vi "GetControlsAndIndicators.vi"(11 "TopLevelDiagram in":refnum<vi>) -> (2 "All Indicators":refnum<vi>[](array[refnum]), 3 "All ControlsTerminals":refnum<vi>[](array[refnum]))   [LabVIEW 2017]
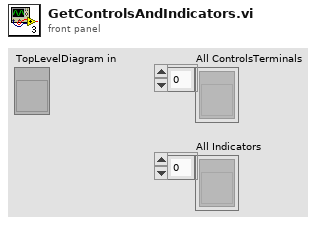
[diagram p1: front panel]
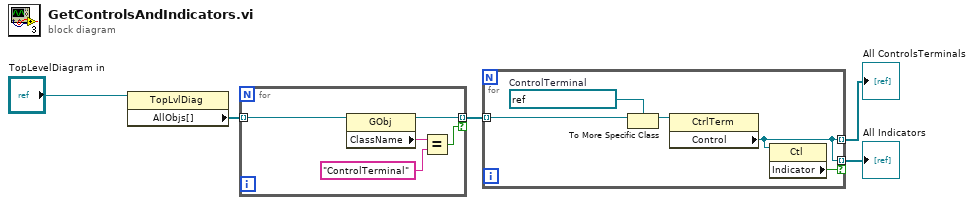
[diagram p0: block diagram]
diagram:
  n1 = property class="TopLvlDiag"(reference="TopLevelDiagram in") -> ("AllObjs[]"=w2:refnum<vi>[])  [unwired: 1 in, 2 out]
  n2 = for {
    tunnel: w2 -> [w10] mode=indexing
    tunnel: [w9] -> w3 mode=indexing if=w6
    n3 = property class="GObj"(reference=w10) -> (reference out=w9:refnum<vi>, "ClassName"=w8:string)  [unwired: 1 in, 1 out]
    n4 = Equal?(x=w8, y="ControlTerminal") -> (x = y?=w6:bool)
  }
  n5 = for {
    tunnel: w3 -> [w15] mode=indexing
    tunnel: [w12] -> w4 mode=indexing
    tunnel: [w12] -> w5 mode=indexing if=w11
    w14 = refnum<vi> refnum  # ControlTerminal
    n6 = To More Specific Class(target class=w14, reference=w15) -> (specific class reference=w13:refnum<vi>)  [unwired: 1 in, 1 out]
    n7 = property class="CtrlTerm"(reference=w13) -> ("Control"=w12:refnum<vi>)  [unwired: 1 in, 2 out]
    n8 = property class="Ctl"(reference=w12) -> ("Indicator"=w11:bool)  [unwired: 1 in, 2 out]
  }
  "All Indicators" <- w5
  "All ControlsTerminals" <- w4
